vi "Teleop.vi"(10 "Match Info":T1={"Autonomous Elapsed Seconds"=0.0, "TeleOp Elapsed Seconds"=0.0, "Disabled Elapsed Seconds"=0.0, "Visited Autonomous"=FALSE, "Visited TeleOp"=FALSE, "Visited Disabled"=FALSE, "Autonomous Settings"={"Autonomous Style"=enum."Independent", "VI Refnum"=refnum}}, 11 "Call Context":T2) -> ()   [LabVIEW 2016]
doc: "This VI is called for each TeleOp packet received from the DS where the robot is not disabled. It is often used to read from the joysticks and update I/O or to update setpoints for timed control loops. It should complete and return within 20 milliseconds or it may miss DS packets."
uses:
  <vilib>/Rock Robotics/WPI/DriverStation/WPI_DriverStationDerivedRobotMode.ctl
  <vilib>/Rock Robotics/WPI/DriverStation/WPI_DriverStationMatch Info.ctl
  <vilib>/Rock Robotics/Network Tables/NT Read Boolean.vi
  <vilib>/Rock Robotics/Network Tables/NT Read Number.vi
  <vilib>/Rock Robotics/WPI/Utilities/WPI_GetSetVariantRefNum.vi
  <vilib>/Rock Robotics/Network Tables/NT Write Numeric Array.vi
  <vilib>/Rock Robotics/Network Tables/NT Write Boolean Array.vi
panel:
  out "y":dbl
  out "x":dbl
  out "Test2":dbl
  out "Test1":dbl
  out "Test Button 2":dbl
  out "Test Button 1":dbl
  out "Lift Bottom":dbl
  out "Lift Top":dbl
  out "Sample Slider 0":dbl(slide) scale=0.0..5.0
  out "Sample Boolean 1":bool
  out "Sample Boolean 0":bool
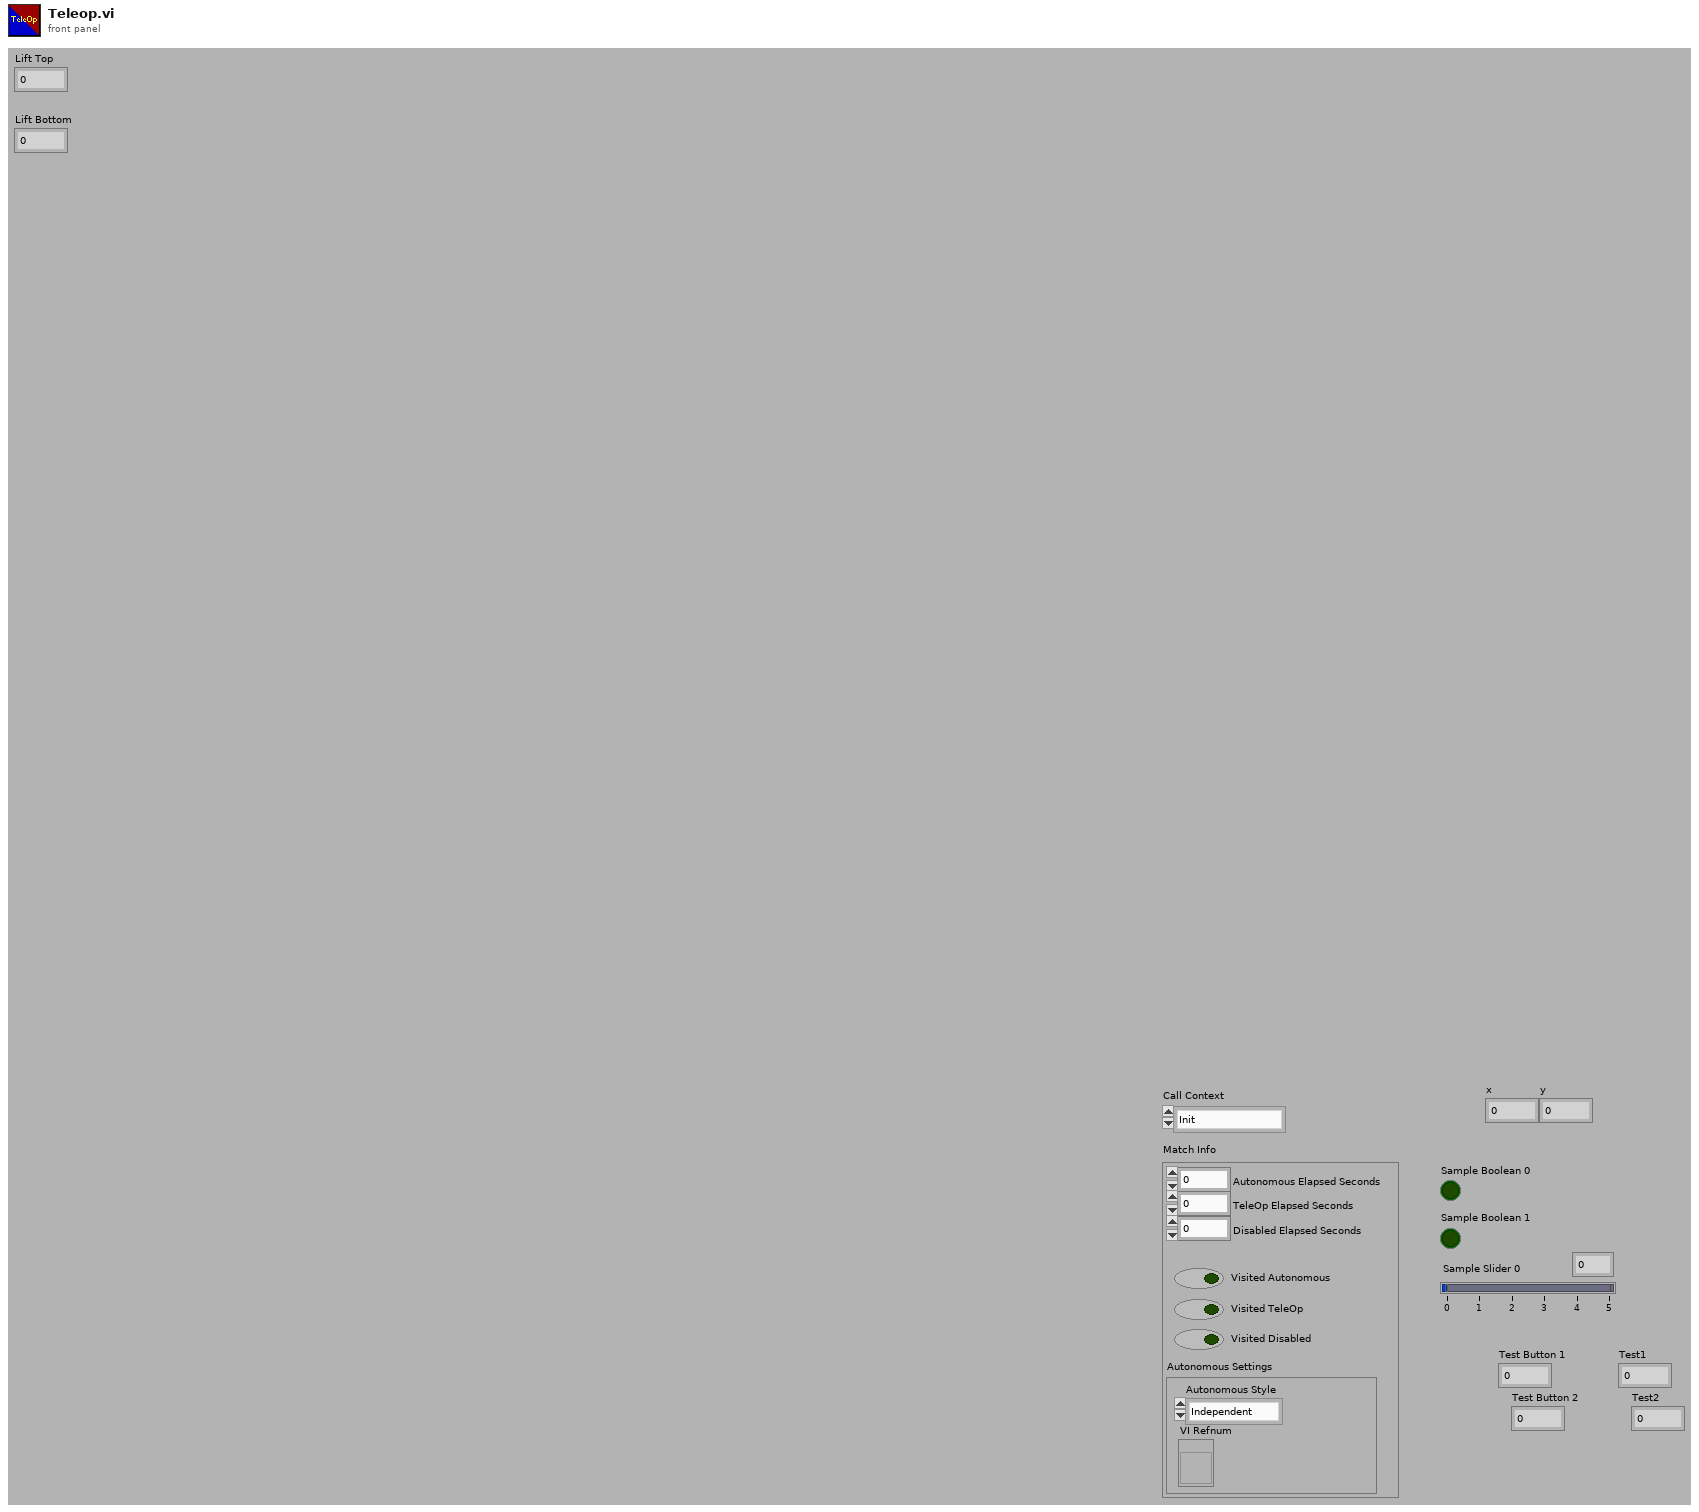
[diagram p1: front panel]
types:
  T1 = typedef "WPI_DriverStationMatch Info.ctl" = cluster{"Autonomous Elapsed Seconds":dbl, "TeleOp Elapsed Seconds":dbl, "Disabled Elapsed Seconds":dbl, "Visited Autonomous":bool, "Visited TeleOp":bool, "Visited Disabled":bool, "Autonomous Settings":cluster{"Autonomous Style":enum16{"Iterative", "Independent"}, "VI Refnum":refnum<vi>}}
  T2 = typedef "WPI_DriverStationDerivedRobotMode.ctl" = enum16{"Init", "Execute", "Stop"}
  T3 = typedef "WPI_JoystickDevRef.ctl" = cluster{"Device":T4}
  T4 = typedef "WPI_JoystickDeviceEnum.ctl" = enum16{"USB 0", "USB 1", "USB 2", "USB 3", "USB 4", "USB 5"}
  T5 = typedef "WPI_ServoDeviceRef.ctl" = cluster{"DeviceStatus":errorcluster, "PWM Channel":T6, "DeadBand":T7}
  T6 = typedef "FPGA_DIOPWMChannel.ctl" = enum8{"PWM 0", "PWM 1", "PWM 2", "PWM 3", "PWM 4", "PWM 5", "PWM 6", "PWM 7", "PWM 8", "PWM 9", "PWM MXP 0", "PWM MXP 1", "PWM MXP 2", "PWM MXP 3", "PWM MXP 4", "PWM MXP 5", "PWM MXP 6", "PWM MXP 7", "PWM MXP 8", "PWM MXP 9", "Invalid"}
  T7 = typedef "WPI_PWMDeadband.ctl" = cluster{"Name":string, "maxPositivePwm":i32, "minPositivePwm":i32, "centerPwm":i32, "maxNegativePwm":i32, "minNegativePwm":i32, "angularRange":u16}
  T8 = typedef "WPI_DigitalInputDevRef.ctl" = cluster{"DevStatus":errorcluster, "DIO Channel":T9}
  T9 = typedef "FPGA_DIOChannel.ctl" = enum8{"DIO 0", "DIO 1", "DIO 2", "DIO 3", "DIO 4", "DIO 5", "DIO 6", "DIO 7", "DIO 8", "DIO 9", "DIO MXP 0", "DIO MXP 1", "DIO MXP 2", "DIO MXP 3", "DIO MXP 4", "DIO MXP 5", "DIO MXP 6", "DIO MXP 7", "DIO MXP 8", "DIO MXP 9", "DIO MXP 10", "DIO MXP 11", "DIO MXP 12", "DIO MXP 13", "DIO MXP 14", "DIO MXP 15", "SPI Port CS1", "SPI Port CS2", "SPI Port CS3", "SPI Port MISO", "SPI Port MOSI", "Invalid"}
  T10 = cluster{"Axes[0]":dbl, "Axes[1]":dbl, "Axes[2]":dbl, "Axes[3]":dbl, "Axes[4]":dbl, "Axes[5]":dbl, "Axes[6]":dbl, "Axes[7]":dbl, "Axes[8]":dbl}
  T11 = cluster{"Buttons[0]":bool, "Buttons[1]":bool, "Buttons[2]":bool, "Buttons[3]":bool, "Buttons[4]":bool, "Buttons[5]":bool, "Buttons[6]":bool, "Buttons[7]":bool, "Buttons[8]":bool}
  T12 = typedef "WPI_MotorControlDeviceRef.ctl" = cluster{"DeviceStatus":errorcluster, "Type":T13, "PWM":cluster{"PWM Channel":T6, "DeadBand":T7}, "CAN":cluster{"Device Number":u8, "SetOutput VI Ref":variant, "GetOutput VI Ref":variant, "Enable VI Ref":variant, "Disable VI Ref":variant, "Data":variant}, "Invert":bool}
  T13 = typedef "WPI_MotorControlType.ctl" = enum16{"PWM", "CAN"}
  T14 = typedef "WPI_RobotDriveDevRef.ctl" = cluster{"DevStatus":errorcluster, "Motors[]":T12[], "Square Inputs":bool, "Max Output":dbl}
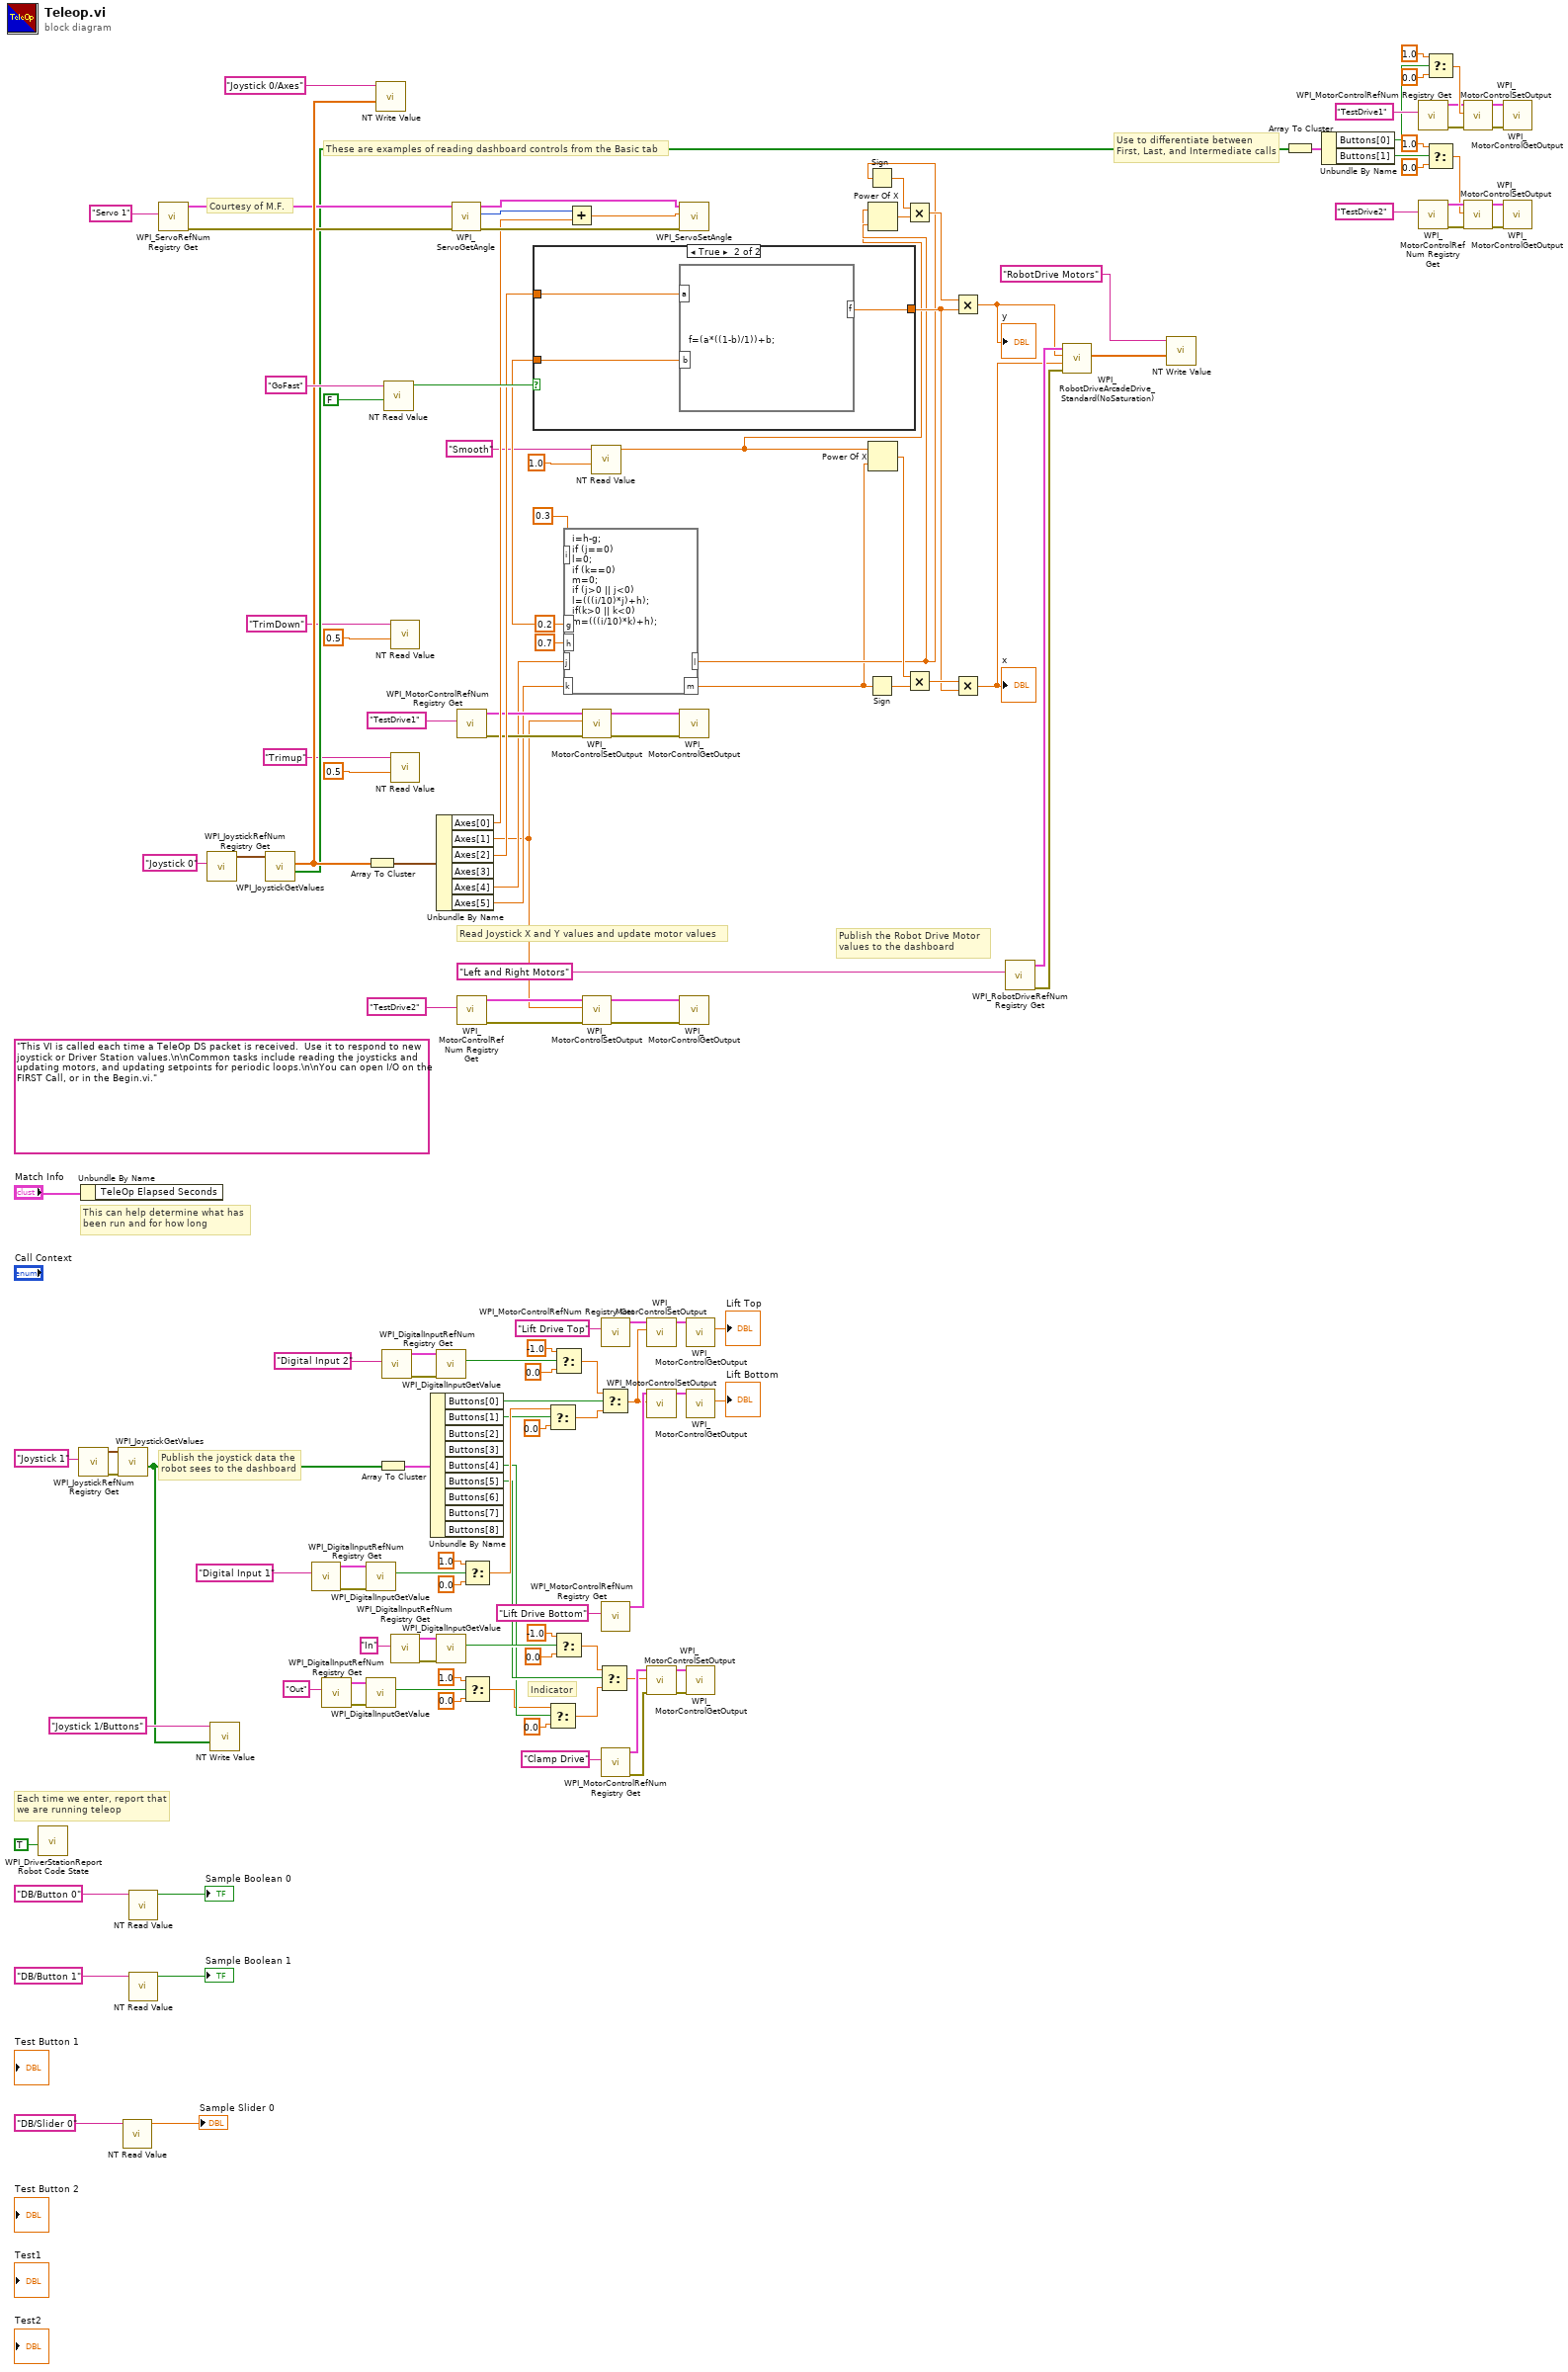
[diagram p0: block diagram]
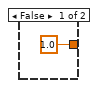
[diagram p2: hidden frame]
diagram:
  w17 = 0.2 ("input variable")
  (unwired) "This VI is called each time a TeleOp DS packet is received.  Use it to respond to new joystick or Driver Station values.\n\nCommon tasks include reading the joysticks and updating motors, and updating setpoints for periodic loops.\n\nYou can open I/O on the FIRST Call, or in the Begin.vi."
  # "Courtesy of M.F."
  # "Indicator"
  # "Publish the Robot Drive Motor\nvalues to the dashboard"
  # "Publish the joystick data the\nrobot sees to the dashboard"
  # "Read Joystick X and Y values and update motor values"
  # "These are examples of reading dashboard controls from the Basic tab"
  # "Each time we enter, report that\nwe are running teleop"
  # "Use to differentiate between\nFirst, Last, and Intermediate calls"
  # "This can help determine what has\nbeen run and for how long"
  n1 = call <vilib>:"WPI_DriverStationReport Robot Code State.vi"("TeleOp"=TRUE ("Autonomous")) -> ()  [unwired: 10 in, 1 out]
  n2 = call <vilib>:"WPI_JoystickRefNum Registry Get.vi"("refnum name"="Joystick 1") -> ("error out"=w56:errorcluster, "JoystickDevRef"=w100:T3)  [unwired: 9 in]
  n3 = Unbundle By Name("Match Info") -> ()  [unwired: 1 out]
  n4 = call <vilib>:"WPI_JoystickGetValues.vi"("error in (no error)"=w56, "JoystickDevRef"=w100) -> ("Buttons"=w99:bool[])  [unwired: 5 in, 4 out]
  n5 = call-poly <vilib>:"NT Read Value.vi"("Name"="DB/Slider 0" ("refnum name")) -> ("Numeric"=→"Sample Slider 0":dbl)  [unwired: 9 in, 1 out]
  n6 = call-poly <vilib>:"NT Read Value.vi"("Name"="DB/Button 0" ("refnum name")) -> ("Boolean"=→"Sample Boolean 0":bool)  [unwired: 9 in, 1 out]
  n7 = call-poly <vilib>:"NT Read Value.vi"("Name"="DB/Button 1" ("refnum name")) -> ("Boolean"=→"Sample Boolean 1":bool)  [unwired: 9 in, 1 out]
  n8 = call <vilib>:"WPI_ServoRefNum Registry Get.vi"("refnum name"="Servo 1") -> ("error out"=w60:errorcluster, "ServoDeviceRef"=w61:T5)  [unwired: 9 in]
  n9 = call <vilib>:"WPI_JoystickRefNum Registry Get.vi"("refnum name"="Joystick 0") -> ("JoystickDevRef"=w131:T3)  [unwired: 1 in, 9 out]
  n10 = call-poly <vilib>:"NT Write Value.vi"("Boolean Array"=w99, "Name"="Joystick 1/Buttons") -> ()  [unwired: 9 in, 1 out]
  n11 = call <vilib>:"WPI_JoystickGetValues.vi"("JoystickDevRef"=w131) -> ("Buttons"=w33:bool[], "Axes"=w108:dbl[])  [unwired: 6 in, 3 out]
  n12 = call <vilib>:"WPI_DigitalInputRefNum Registry Get.vi"("refnum name"="Digital Input 1") -> ("error out"=w81:errorcluster, "DigitalInputDevRef"=w82:T8)  [unwired: 9 in]
  n13 = call <vilib>:"WPI_DigitalInputRefNum Registry Get.vi"("refnum name"="Out") -> ("error out"=w65:errorcluster, "DigitalInputDevRef"=w74:T8)  [unwired: 9 in]
  n14 = call <vilib>:"WPI_DigitalInputGetValue.vi"("error in (no error)"=w81, "DigitalInputDevRef"=w82) -> ("Value"=w80:bool)  [unwired: 7 in, 2 out]
  n15 = call <vilib>:"WPI_DigitalInputGetValue.vi"("error in (no error)"=w65, "DigitalInputDevRef"=w74) -> ("Value"=w72:bool)  [unwired: 7 in, 2 out]
  n16 = Array To Cluster(array=w108) -> (cluster=w107:T10)
  n17 = call-poly <vilib>:"NT Write Value.vi"("Numeric Array"=w108, "Name"="Joystick 0/Axes") -> ()  [unwired: 9 in, 1 out]
  n18 = Array To Cluster(array=w99) -> (cluster=w109:T11)
  n19 = call <vilib>:"WPI_DigitalInputRefNum Registry Get.vi"("refnum name"="Digital Input 2") -> ("error out"=w85:errorcluster, "DigitalInputDevRef"=w86:T8)  [unwired: 9 in]
  n20 = call-poly <vilib>:"NT Read Value.vi"("Default Value"=FALSE, "Name"="GoFast" ("refnum name")) -> ("Boolean"=w104:bool)  [unwired: 8 in, 1 out]
  n21 = call-poly <vilib>:"NT Read Value.vi"("Default Value"=0.5, "Name"="TrimDown" ("refnum name")) -> ()  [unwired: 8 in, 2 out]
  n22 = call-poly <vilib>:"NT Read Value.vi"("Default Value"=0.5, "Name"="Trimup" ("refnum name")) -> ()  [unwired: 8 in, 2 out]
  n23 = call <vilib>:"WPI_DigitalInputRefNum Registry Get.vi"("refnum name"="In") -> ("error out"=w96:errorcluster, "DigitalInputDevRef"=w98:T8)  [unwired: 9 in]
  n24 = Unbundle By Name(w109) -> ("Buttons[0]"=w101:bool, "Buttons[1]"=w78:bool, "Buttons[4]"=w75:bool, "Buttons[5]"=w77:bool)  [unwired: 5 out]
  n25 = Unbundle By Name(w107) -> ("Axes[0]"=w55:dbl, "Axes[1]"=w14:dbl, "Axes[2]"=w102:dbl, "Axes[4]"=w19:dbl, "Axes[5]"=w18:dbl)  [unwired: 1 out]
  n26 = call <vilib>:"WPI_DigitalInputGetValue.vi"("error in (no error)"=w85, "DigitalInputDevRef"=w86) -> ("Value"=w84:bool)  [unwired: 7 in, 2 out]
  n27 = call <vilib>:"WPI_DigitalInputGetValue.vi"("error in (no error)"=w96, "DigitalInputDevRef"=w98) -> ("Value"=w94:bool)  [unwired: 7 in, 2 out]
  n28 = call <vilib>:"WPI_ServoGetAngle.vi"("ServoDeviceRef"=w61, "error in (no error)"=w60) -> ("ServoDeviceRef"=w58:T5, "Angle"=w63:u16, "error out"=w59:errorcluster)  [unwired: 6 in]
  n29 = call <vilib>:"WPI_MotorControlRefNum Registry Get.vi"("refnum name"="TestDrive1") -> ("error out"=w48:errorcluster, "MotorControlDevRef"=w54:T12)  [unwired: 9 in]
  n30 = call <vilib>:"WPI_MotorControlRefNum Registry Get.vi"("refnum name"="TestDrive2") -> ("error out"=w47:errorcluster, "MotorControlDevRef"=w51:T12)  [unwired: 9 in]
  n31 = Select(t=1.0, s=w80, f=0.0) -> (s? t:f=w91:dbl)
  n32 = Select(t=1.0, s=w72, f=0.0) -> (s? t:f=w69:dbl)
  n33 = case shown="True" w104 {
    tunnel: [1.0 ("f") w143] -> w10
    tunnel: w17 -> [_ w144]
    tunnel: w102 -> [_ w145]
    frame False {
    }
    frame True {
      n34 = formula code="f=(a*((1-b)/1))+b;"("a"=w145, "b"=w144) -> ("f"=w143:dbl)
    }
  }
  n35 = Select(t=w91, s=w78, f=0.0) -> (s? t:f=w115:dbl)
  n36 = Select(t=w69, s=w75, f=0.0) -> (s? t:f=w66:dbl)
  n37 = Select(t=-1.0, s=w84, f=0.0) -> (s? t:f=w92:dbl)
  n38 = Select(t=-1.0, s=w94, f=0.0) -> (s? t:f=w67:dbl)
  n39 = formula code="i=h-g;\nif (j==0)\nl=0;\nif (k==0)\nm=0;\nif (j>0 || j<0)\nl=(((i/10)*j)+h);\nif(k>0 || k<0)\nm=(((i/10)*k)+h);"("g"=w17, "h"=0.7 ("input variable"), "j"=w19, "k"=w18, "i"=0.3 ("input variable")) -> ("l"=w6:dbl, "m"=w5:dbl)
  n40 = Add(x=w63, y=w55) -> (x+y=w64:dbl)
  n41 = call <vilib>:"WPI_MotorControlSetOutput.vi"("error in (no error)"=w48, "Output"=w14, "MotorControlDevRef"=w54) -> ("error out"=w46:errorcluster, "MotorControlDevRef"=w50:T12)  [unwired: 6 in, 1 out]
  n42 = call <vilib>:"WPI_MotorControlSetOutput.vi"("error in (no error)"=w47, "Output"=w14, "MotorControlDevRef"=w51) -> ("error out"=w45:errorcluster, "MotorControlDevRef"=w49:T12)  [unwired: 6 in, 1 out]
  n43 = call-poly <vilib>:"NT Read Value.vi"("Default Value"=1.0, "Name"="Smooth") -> ("Numeric"=w3:dbl)  [unwired: 8 in, 1 out]
  n44 = Select(t=w67, s=w77, f=w66) -> (s? t:f=w93:dbl)
  n45 = call <vilib>:"WPI_MotorControlRefNum Registry Get.vi"("refnum name"="Lift Drive Top") -> ("MotorControlDevRef"=w122:T12)  [unwired: 9 in, 1 out]
  n46 = Select(t=w92, s=w101, f=w115) -> (s? t:f=w116:dbl)
  n47 = call <vilib>:"WPI_MotorControlRefNum Registry Get.vi"("refnum name"="Lift Drive Bottom") -> ("MotorControlDevRef"=w121:T12)  [unwired: 9 in, 1 out]
  n48 = call <vilib>:"WPI_MotorControlRefNum Registry Get.vi"("refnum name"="Clamp Drive") -> ("error out"=w114:errorcluster, "MotorControlDevRef"=w112:T12)  [unwired: 9 in]
  n49 = call <vilib>:"WPI_MotorControlSetOutput.vi"("Output"=w116, "MotorControlDevRef"=w122) -> ("MotorControlDevRef"=w123:T12)  [unwired: 7 in, 2 out]
  n50 = call <vilib>:"WPI_MotorControlSetOutput.vi"("Output"=w116, "MotorControlDevRef"=w121) -> ("MotorControlDevRef"=w124:T12)  [unwired: 7 in, 2 out]
  n51 = call <vilib>:"WPI_MotorControlSetOutput.vi"("error in (no error)"=w114, "Output"=w93, "MotorControlDevRef"=w112) -> ("error out"=w111:errorcluster, "MotorControlDevRef"=w113:T12)  [unwired: 6 in, 1 out]
  n52 = call <vilib>:"WPI_ServoSetAngle.vi"("error in (no error)"=w59, "Angle"=w64, "ServoDeviceRef"=w58) -> ()  [unwired: 7 in, 2 out]
  n53 = call <vilib>:"WPI_MotorControlGetOutput.vi"("error in"=w46, "MotorControlDevRef"=w50) -> ()  [unwired: 7 in, 3 out]
  n54 = call <vilib>:"WPI_MotorControlGetOutput.vi"("error in"=w45, "MotorControlDevRef"=w49) -> ()  [unwired: 7 in, 3 out]
  n55 = call <vilib>:"WPI_MotorControlGetOutput.vi"("MotorControlDevRef"=w123) -> ("Output"=→"Lift Top":dbl)  [unwired: 8 in, 2 out]
  n56 = call <vilib>:"WPI_MotorControlGetOutput.vi"("MotorControlDevRef"=w124) -> ("Output"=→"Lift Bottom":dbl)  [unwired: 8 in, 2 out]
  n57 = call <vilib>:"WPI_MotorControlGetOutput.vi"("error in"=w111, "MotorControlDevRef"=w113) -> ()  [unwired: 7 in, 3 out]
  n58 = Sign(1:w6) -> (0:w12:dbl)
  n59 = Sign(1:w5) -> (0:w9:dbl)
  n60 = Power Of X(1:w6, 2:w3) -> (0:w7:dbl)
  n61 = Power Of X(1:w5, 2:w3) -> (0:w8:dbl)
  n62 = Multiply(x=w12, y=w7) -> (x*y=w13:dbl)
  n63 = Multiply(x=w8, y=w9) -> (x*y=w11:dbl)
  n64 = Multiply(x=w13, y=w10) -> (x*y=w16:dbl)
  "y" <- w16
  n65 = Multiply(x=w11, y=w10) -> (x*y=w15:dbl)
  "x" <- w15
  n66 = call <vilib>:"WPI_RobotDriveRefNum Registry Get.vi"("refnum name"="Left and Right Motors") -> ("error out"=w106:errorcluster, "RobotDriveDevRef"=w132:T14)  [unwired: 1 in, 8 out]
  n67 = call <vilib>:"WPI_RobotDriveArcadeDrive_Standard(NoSaturation).vi"("error in (no error)"=w106, "Y axis value"=w15, "X axis value"=w16, "RobotDriveDevRef"=w132) -> ("Motor Values"=w127:dbl[])  [unwired: 7 out]
  n68 = call-poly <vilib>:"NT Write Value.vi"("Numeric Array"=w127, "Name"="RobotDrive Motors") -> ()  [unwired: 9 in, 1 out]
  n69 = Array To Cluster(array=w33) -> (cluster=w31:T11)
  n70 = Unbundle By Name(w31) -> ("Buttons[0]"=w30:bool, "Buttons[1]"=w29:bool)
  n71 = call <vilib>:"WPI_MotorControlRefNum Registry Get.vi"("refnum name"="TestDrive1") -> ("error out"=w26:errorcluster, "MotorControlDevRef"=w27:T12)  [unwired: 9 in]
  n72 = call <vilib>:"WPI_MotorControlRefNum Registry Get.vi"("refnum name"="TestDrive2") -> ("error out"=w40:errorcluster, "MotorControlDevRef"=w42:T12)  [unwired: 9 in]
  n73 = Select(t=1.0, s=w30, f=0.0) -> (s? t:f=w28:dbl)
  n74 = Select(t=1.0, s=w29, f=0.0) -> (s? t:f=w36:dbl)
  n75 = call <vilib>:"WPI_MotorControlSetOutput.vi"("error in (no error)"=w26, "Output"=w28, "MotorControlDevRef"=w27) -> ("error out"=w25:errorcluster, "MotorControlDevRef"=w32:T12)  [unwired: 6 in, 1 out]
  n76 = call <vilib>:"WPI_MotorControlSetOutput.vi"("error in (no error)"=w40, "Output"=w36, "MotorControlDevRef"=w42) -> ("error out"=w39:errorcluster, "MotorControlDevRef"=w41:T12)  [unwired: 6 in, 1 out]
  n77 = call <vilib>:"WPI_MotorControlGetOutput.vi"("error in"=w25, "MotorControlDevRef"=w32) -> ()  [unwired: 7 in, 3 out]
  n78 = call <vilib>:"WPI_MotorControlGetOutput.vi"("error in"=w39, "MotorControlDevRef"=w41) -> ()  [unwired: 7 in, 3 out]
